vi "PreSpectraDe-meanAndHalveEnds.vi"(11 "Array":dbl[](array[numeric])) -> (0 "length":i32, 3 "PreppedArray":dbl[](array[numeric]))   [LabVIEW 2020]
doc: "Subtracts the mean from the signal, and halves the first and last values, Used prior to performing Power Spectrum.\nVI is configured \"Inline\", meaning it performs the same as if it was on its parent diagram."
uses:
  <vilib>/Analysis/baseanly.llb/Mean (DBL).vi
  <vilib>/Analysis/NI_AALBase.lvlib
panel:
  out "mean":dbl format="%.2f"
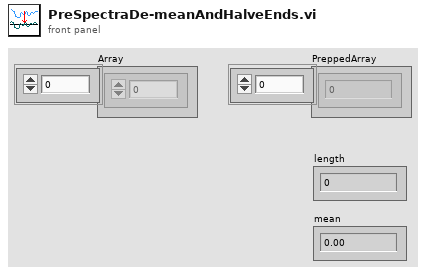
[diagram p1: front panel]
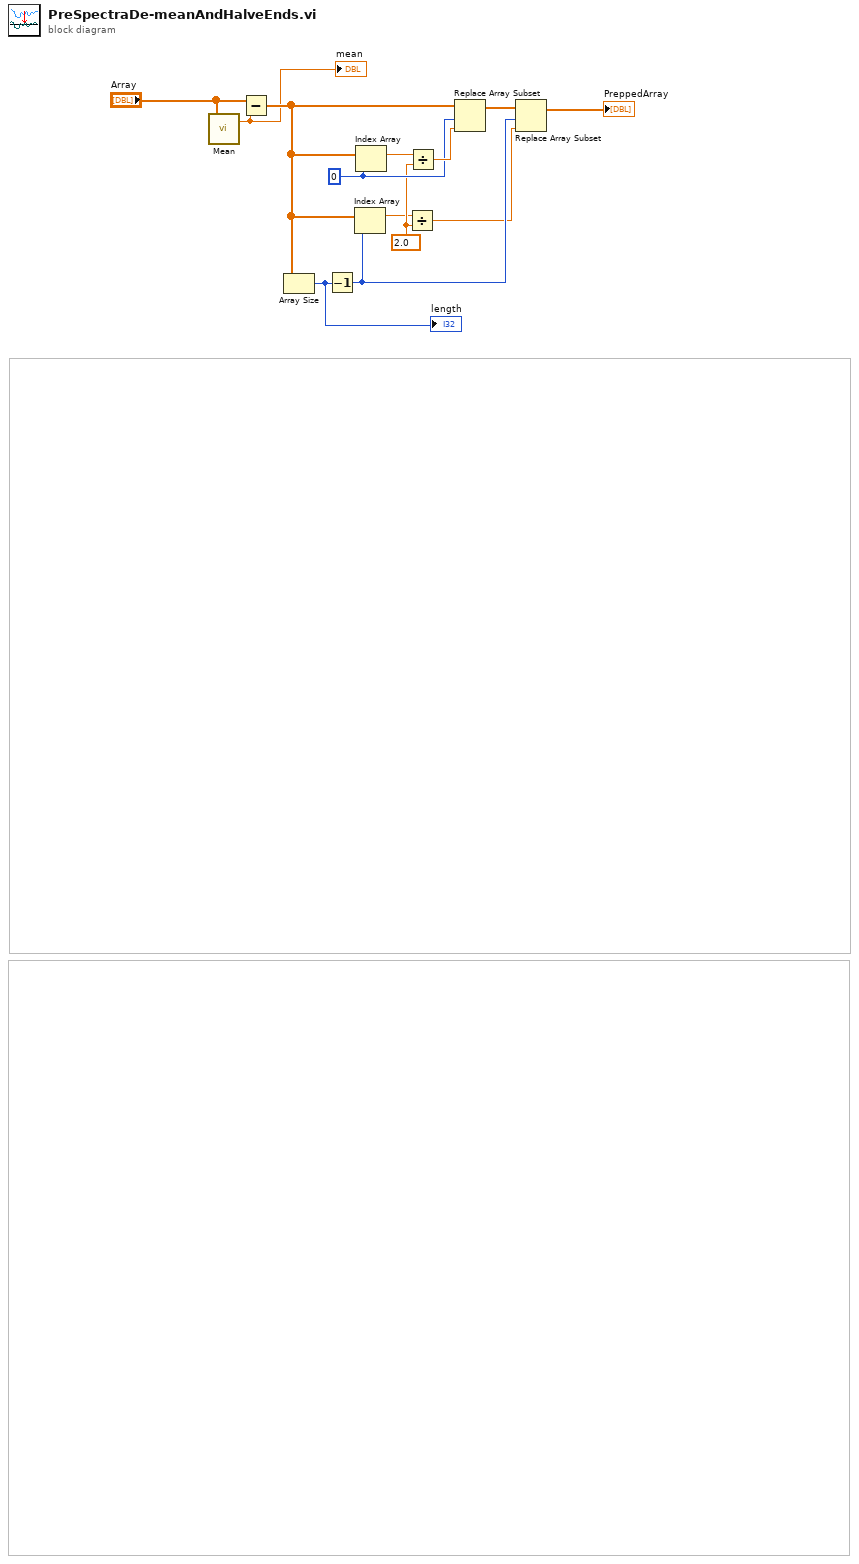
[diagram p0: block diagram]
diagram:
  w6 = 0
  w5 = 2.0
  n1 = call-poly <vilib>:"Mean.vi"("X"="Array") -> ("mean"=w1:dbl)  [unwired: 1 out]
  "mean" <- w1
  n2 = Subtract(x="Array", y=w1) -> (x-y=w13:dbl[])
  n3 = Array Size(array=w13) -> (size(s)=w12:i32)
  "length" <- w12
  n4 = Decrement(x=w12) -> (x-1=w9:i32)
  n5 = Index Array(array=w13, index=w9) -> (element=w4:dbl)
  n6 = Index Array(array=w13, index=w6) -> (element=w3:dbl)
  n7 = Divide(x=w4, y=w5) -> (x/y=w8:dbl)
  n8 = Divide(x=w3, y=w5) -> (x/y=w7:dbl)
  n9 = Replace Array Subset(array=w13, new element=w7, index=w6) -> (w2:dbl[])
  n10 = Replace Array Subset(array=w2, new element=w8, index=w9) -> (→"PreppedArray":dbl[])
